vi "testGetSpecificElement.vi"(8 "error in (no error)":errorcluster) -> (0 "error out":errorcluster)   [LabVIEW 2018]
uses:
  SALTypeGenerator/Topic/Topic.lvclass
  SALTypeGenerator/Element/Element.lvclass
  SALTypeGenerator/Element/Element.lvclass/Element.ctl
  SALTypeGenerator/Topic/Topic.lvclass/Topic.ctl
  <vilib>/addons/_JKI Toolkits/Caraya/classes/Assert/Assert Equal Value_Variant.vi
  <vilib>/addons/_JKI Toolkits/Caraya/classes/Test/Test.lvclass
  <vilib>/addons/_JKI Toolkits/Caraya/classes/Assert/Assert.lvclass
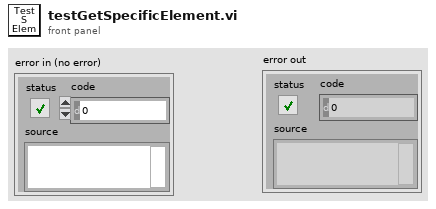
[diagram p1: front panel]
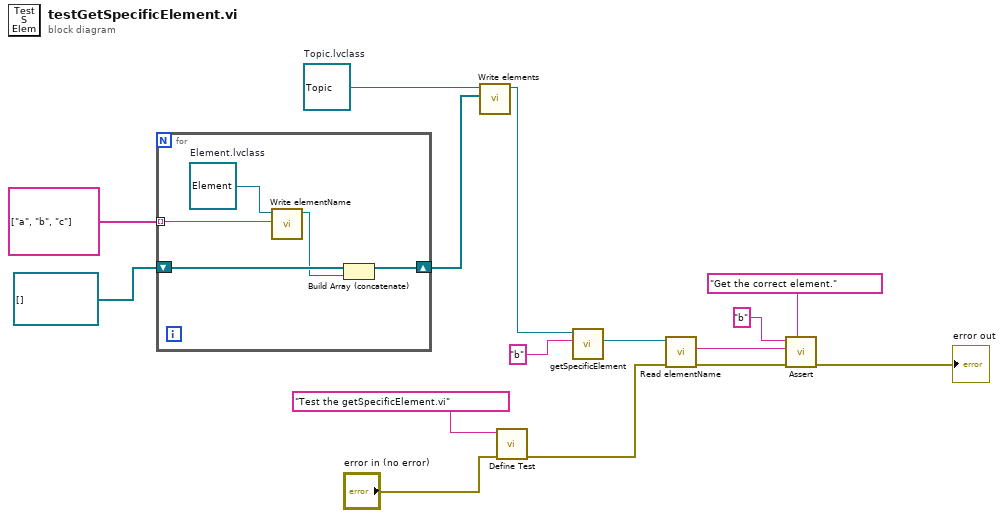
[diagram p0: block diagram]
diagram:
  w15 = refnum<class "Topic.lvclass"> refnum  # Topic.lvclass
  n1 = for {
    tunnel: string[] ["a", "b", "c"] -> [w19] mode=indexing
    shift-right: [w17] -> w12
    shift-left: refnum<class "Element.lvclass">[] [] -> [w18]
    w20 = refnum<class "Element.lvclass"> refnum  # Element.lvclass
    n2 = call "Write elementName.vi"("elementName"=w19, "Element in"=w20) -> ("Element out"=w16:refnum<class "Element.lvclass">)  [unwired: 9 in]
    n3 = Build Array (concatenate)(w18, w16) -> (w17:refnum<class "Element.lvclass">[])
  }
  n4 = call "Write elements.vi"("elements"=w12, "Topic in"=w15) -> ("Topic out"=w11:refnum<class "Topic.lvclass">)  [unwired: 8 in, 1 out]
  n5 = call <vilib>:"Define Test.vi"("error in (no error)"="error in (no error)", "Label (VI Title)"="Test the getSpecificElement.vi") -> ("error out"=w6:errorcluster)  [unwired: 9 in]
  n6 = call "getSpecificElement.vi"("nameElem"="b", "Topic in"=w11) -> ("Element.lvclass"=w9:refnum<class "Element.lvclass">)  [unwired: 7 in, 2 out]
  n7 = call "Read elementName.vi"("error in (no error)"=w6, "Element in"=w9) -> ("error out"=w5:errorcluster, "elementName"=w8:string)  [unwired: 7 in, 1 out]
  n8 = call-poly <vilib>:"Assert.vi"("Label"="Get the correct element.", "error in (no error)"=w5, "Y"=w8, "X"="b") -> ("error out"=→"error out":errorcluster)  [unwired: 7 in]
